vi "Add Heartbeat.vi"(8 "Timeout":u16 format="%d ms", 9 "Period":u16 format="%d ms", 10 "Node ID":u8, 11 "CANopen in":refnum<class "CANopen.lvclass">) -> (3 "CANopen out":refnum<class "CANopen.lvclass">)   [LabVIEW 2024, in "canopen.lvlib" / "CANopen.lvclass"]
doc: "Sets the table where the heartbeat watchdog states are stored and updated."
uses:
  CANopen.lvclass
  CANopen.lvclass/CANopen.ctl
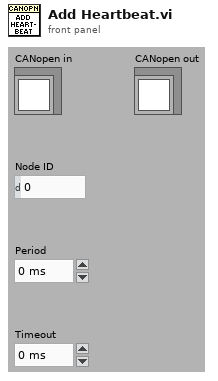
[diagram p1: front panel]
types:
  T1 = cluster{"Period":u16, "Timeout":u16, "Last Beat":timestamp, "Timed Out?":bool}
  T2 = map{u8, cluster{"Period":u16, "Timeout":u16, "Last Beat":timestamp, "Timed Out?":bool}}
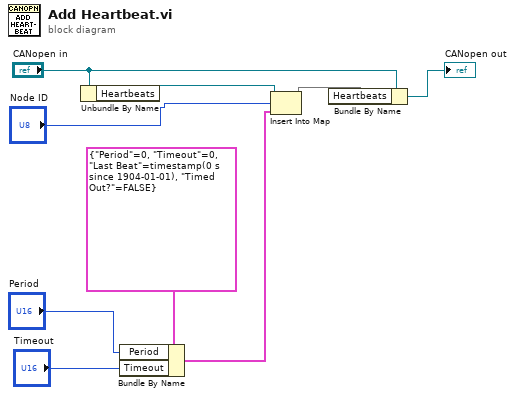
[diagram p0: block diagram]
diagram:
  n1 = Unbundle By Name("CANopen in") -> ("Heartbeats"=w7:refnum<data-value>)
  n2 = Bundle By Name(cluster=T1 {"Period"=0, "Timeout"=0, "Last Beat"=timestamp(0 s since 1904-01-01), "Timed Out?"=FALSE} ("HeartBeatEntry"), "Period"="Period", "Timeout"="Timeout") -> (w3:T1)
  n3 = Insert Into Map(map in=w7, key="Node ID", value=w3) -> (map out=w6:T2)  [unwired: 2 out]
  n4 = Bundle By Name(cluster="CANopen in", "Heartbeats"=w6) -> (→"CANopen out":refnum<class "CANopen.lvclass">)
